vi "Load_XML2.vi"(11 "XML File Path 2":path) -> (3 "DPP Configuration":T1={"reset_recovery_time"=300, "edge_peaking_time"=5, "flat_top"=5, "peaking_time"=25, "gain"=1.0, "max_risetime"=35.0, "fast_filter_thr"=100, "zero_peak_freq"=5.0, "inverted_input"=0, "base_offset"=0, "reset_threshold"=1000, "overflow_recovery"=0, "tail_coefficient"=0.0, "energy_filter_thr"=25, "energy_baseline_thr"=25, "max_peaking_time"=0, "edge_flat_top"=1, "time_constant"=0.0, "baseline_samples"=64, "other_param"=0})   [LabVIEW 2015]
uses:
  ConfigurationDPP.ctl
  <vilib>/xml/Load XML File.vi
  <vilib>/xml/Close Reference(Node).vi
  <resource>/objmgr/DOMUserDefRef.rc
  <vilib>/xml/NI_XML.lvlib
panel:
  out "Parse Errors 2":string
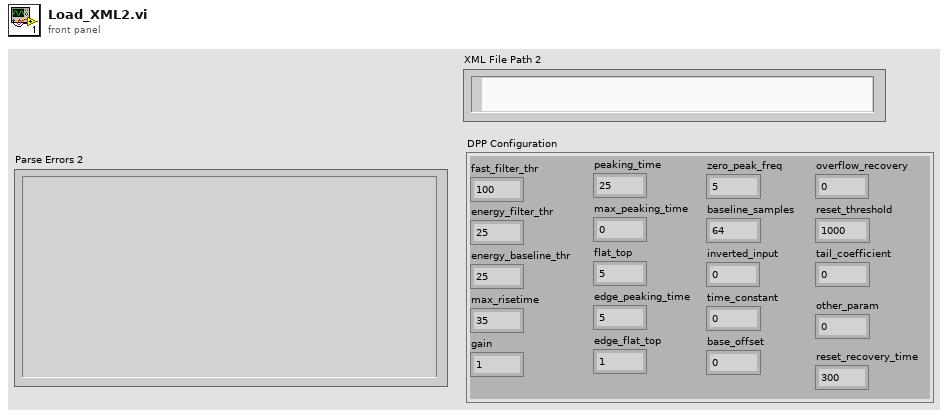
[diagram p1: front panel]
types:
  T1 = typedef "ConfigurationDPP.ctl" = cluster{"reset_recovery_time":u32, "edge_peaking_time":u32, "flat_top":u32, "peaking_time":u32, "gain":dbl, "max_risetime":dbl, "fast_filter_thr":u32, "zero_peak_freq":dbl, "inverted_input":u8, "base_offset":u32, "reset_threshold":u32, "overflow_recovery":u32, "tail_coefficient":dbl, "energy_filter_thr":u32, "energy_baseline_thr":u32, "max_peaking_time":u32, "edge_flat_top":u32, "time_constant":dbl, "baseline_samples":u32, "other_param":u32}
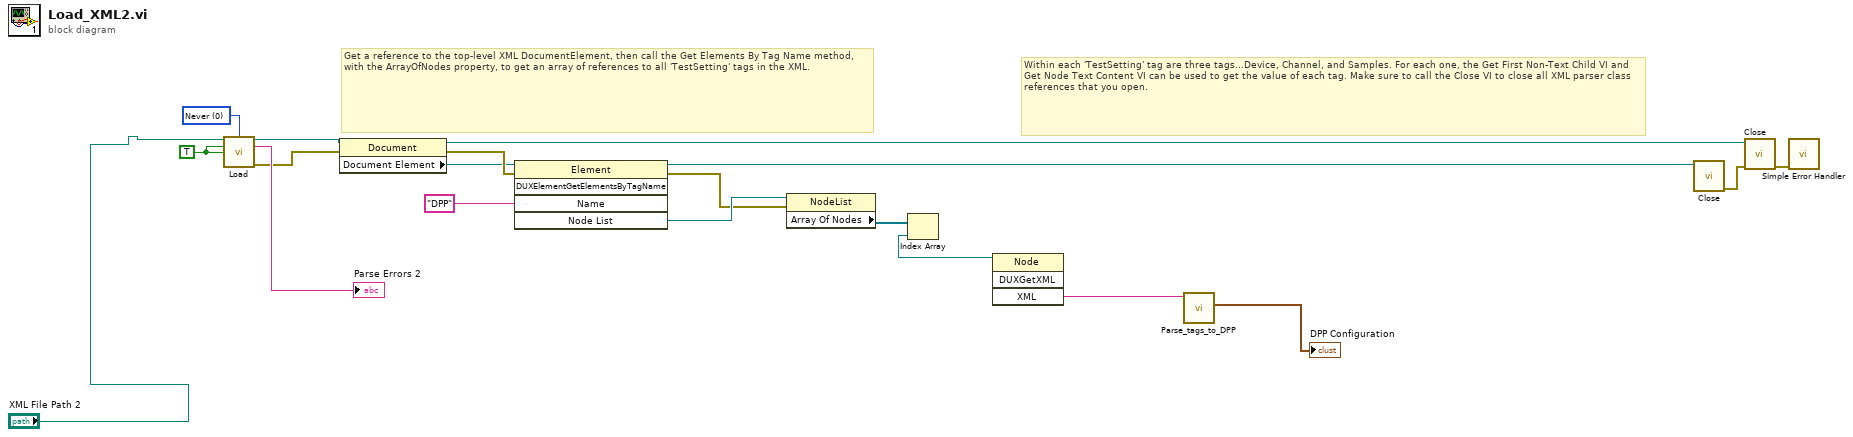
[diagram p0: block diagram]
diagram:
  w19 = 0 items=["Never", "Always", "Auto"] ("Validate On Load")
  w8 = TRUE ("Do Namespaces")
  # "Within each 'TestSetting' tag are three tags...Device, Channel, and Samples. For each one, the Get First Non-Text Child VI and Get Node Text Content VI can be used to get the value of each tag. Make sure to call the Close VI to close all XML parser class references that you open."
  # "Get a reference to the top-level XML DocumentElement, then call the Get Elements By Tag Name method, with the ArrayOfNodes property, to get an array of references to all 'TestSetting' tags in the XML."
  n1 = call-poly <vilib>:"Load.vi"("path to XML document"="XML File Path 2", "validate on load (Auto)"=w19, "process namespaces (False)"=w8, "process schema (False)"=w8) -> ("DOM document out"=w7:refnum<k20>, "parse errors"=→"Parse Errors 2":string, "error out"=w10:errorcluster)  [unwired: 3 in, 6 out]
  n2 = property class="Document"(reference=w7, error in=w10) -> (reference out=w11:refnum<k20>, error out=w16:errorcluster, "Document Element"=w5:refnum<k20>)
  n3 = invoke class="Element" method="DUXElementGetElementsByTagName"(reference=w5, error in=w16, "Name"="DPP" ("Node Name")) -> (reference out=w13:refnum<k20>, error out=w14:errorcluster, "Node List"=w15:refnum<k20>)  [unwired: 2 in, 2 out]
  n4 = property class="NodeList"(reference=w15, error in=w14) -> ("Array Of Nodes"=w4:refnum<k20>[])  [unwired: 2 out]
  n5 = Index Array(array=w4) -> (element=w3:refnum<k20>)  [unwired: 1 in]
  n6 = invoke on="Invoke Node" class="Node" method="DUXGetXML"(reference=w3) -> ("XML"=w2:string)  [unwired: 3 in, 3 out]
  n7 = call "Parse_tags_to_DPP.vi"("XML"=w2) -> ("DPP Configuration"=→"DPP Configuration":T1)  [unwired: 10 in]
  n8 = call-poly <vilib>:"Close.vi"("node"=w13) -> ("error out"=w12:errorcluster)  [unwired: 1 in, 7 out]
  n9 = call-poly <vilib>:"Close.vi"("error in (no error)"=w12, "node"=w11) -> ("error out"=w9:errorcluster)  [unwired: 7 out]
  n10 = call <vilib>:"Simple Error Handler.vi"("error in (no error)"=w9) -> ()  [unwired: 4 in, 5 out]
